vi "StringArrayParsing.vi"(9 "delimiter":string, 10 "Input String":string) -> (0 "#ofPerfectElement":i32, 1 "After":string, 2 "Before":string, 3 "Result":string[](array[string]))   [LabVIEW 2013]
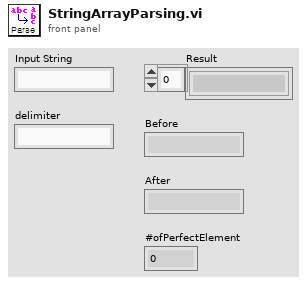
[diagram p1: front panel]
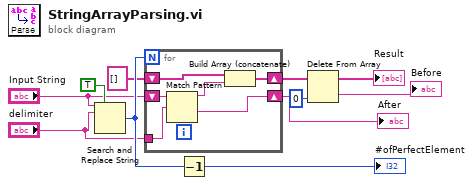
[diagram p0: block diagram]
diagram:
  n1 = Search and Replace String(replace all?=TRUE ("replace all? (F)"), input string="Input String", search string="delimiter") -> (number of replacements=w10:i32)  [unwired: 5 in, 3 out]
  n2 = for {
    N: w10 -> [_]
    shift-right: [w16] -> w3
    shift-left: "Input String" -> [w17]
    shift-right: [w12] -> w4
    shift-left: string[] [] -> [w13]
    tunnel: "delimiter" -> [w15]
    n3 = Match Pattern(string=w17, regular expression=w15) -> (before substring=w14:string, after substring=w16:string)  [unwired: 1 in, 2 out]
    n4 = Build Array (concatenate)(w13, w14) -> (w12:string[])
  }
  "After" <- w3
  n5 = Decrement(x=w10) -> (x-1=→"#ofPerfectElement":i32)
  n6 = Delete From Array(array=w4, index=0) -> (deleted portion=→"Before":string, array with subset deleted=→"Result":string[])  [unwired: 1 in]
